vi "SS Launch GUI Dynamic.vi"(7 "VI Refnum":refnum<vi>, 8 "error in (no error)":errorcluster, 10 "Data":variant, 11 "Device Name":string) -> (0 "error out":errorcluster, 2 "VI Clone Name":string, 3 "reference out":refnum<vi>)   [LabVIEW 2021]
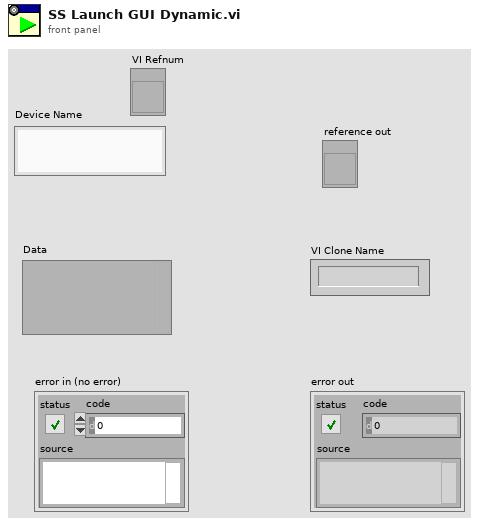
[diagram p1: front panel]
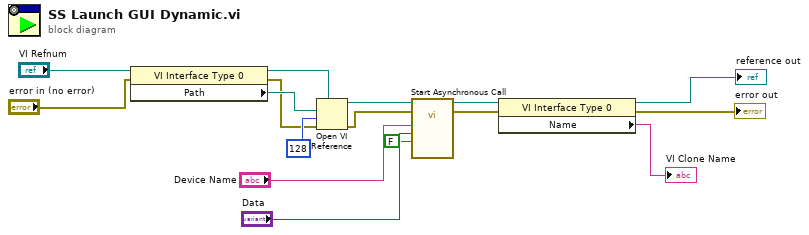
[diagram p0: block diagram]
diagram:
  n1 = property class="VI Interface Type 0"(reference="VI Refnum", error in="error in (no error)") -> (reference out=w7:refnum<vi>, error out=w3:errorcluster, "Path"=w8:path)
  n2 = Open VI Reference(type specifier VI Refnum (for type only)=w7, vi path=w8, options=128, error in (no error)=w3) -> (vi reference=w15:refnum<vi>, error out=w14:errorcluster)  [unwired: 2 in]
  n3 = call-by-ref "Start Asynchronous Call"(reference=w15, error in=w14, "Standalone"=FALSE, "Init Data"="Data", "Filter Wheel name"="Device Name") -> (reference out=w13:refnum<vi>, error out=w12:errorcluster)  [unwired: 9 in]
  n4 = property class="VI Interface Type 0"(reference=w13, error in=w12) -> (reference out=→"reference out":refnum<vi>, error out=→"error out":errorcluster, "Name"=→"VI Clone Name":string)
